vi "ARN Name fuer Datei.vi"(11 "String Eingabe":T1) -> (3 "File Name":string)   [LabVIEW 2020, in "EPA 1065.lvlib" / "ARN Test 1065-305.lvlib"]
uses:
  ARN Test 1065-305.lvlib
  Visualisierungs Elemente/String - Eingabefeld.ctl
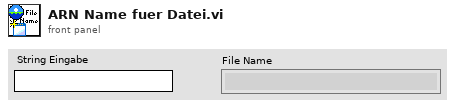
[diagram p1: front panel]
types:
  T1 = typedef "String - Eingabefeld.ctl" = string
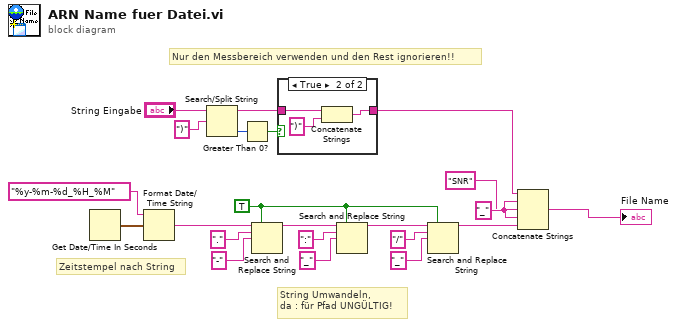
[diagram p0: block diagram]
diagram:
  w3 = "_"
  w14 = TRUE ("Alle ersetzen? (F)")
  # "Nur den Messbereich verwenden und den Rest ignorieren!!"
  # "String Umwandeln, \nda : für Pfad UNGÜLTIG!"
  # "Zeitstempel nach String"
  n1 = Get Date/Time In Seconds() -> (seconds since 1Jan1904=w4:timestamp)
  n2 = Format Date/Time String(time format string (%c)="%y-%m-%d_%H_%M" ("Zeitformatierungs-String (%c)"), seconds (now)=w4) -> (date/time string=w5:string)  [unwired: 1 in]
  n3 = Search/Split String(string="String Eingabe", search string/char (-)=")" ("Nach String/Zeichen suchen (-)")) -> (substring before match=w21:T1, offset of match=w19:i32)  [unwired: 1 in, 1 out]
  n4 = Greater Than 0?(x=w19) -> (x > 0?=w20:bool)
  n5 = Search and Replace String(replace all?=w14, input string=w5, search string="." ("Such-String"), replace string="-" ("String ersetzen(\"\")")) -> (result string=w8:string)  [unwired: 4 in, 3 out]
  n6 = case shown="True" w20 {
    tunnel: w21 -> [w23 w26]
    tunnel: [w23 w25] -> w2
    frame False {
    }
    frame True {
      n7 = Concatenate Strings(w26, ")" ("String")) -> (w25:string)
    }
  }
  n8 = Search and Replace String(replace all?=w14, input string=w8, search string=":" ("Such-String"), replace string="_" ("String ersetzen(\"\")")) -> (result string=w13:string)  [unwired: 4 in, 3 out]
  n9 = Search and Replace String(replace all?=w14, input string=w13, search string="/" ("Such-String"), replace string="_" ("String ersetzen(\"\")")) -> (result string=w15:string)  [unwired: 4 in, 3 out]
  n10 = Concatenate Strings(w2, w3, T1 "SNR" ("String"), w3, w15) -> (→"File Name":string)
